vi "solar_cfg Write (Str).vi"(0 "Config Refnum":refnum<data-value>, 1 "Section":string, 2 "Comment":string, 5 "Key":string, 7 "Value in":string, 9 "Add Quotes? (T)":bool=TRUE, 11 "error in (no error)":errorcluster) -> (4 "dup Config Refnum":refnum<data-value>, 10 "Found?":bool, 15 "error out":errorcluster)   [LabVIEW 2018]
doc: "Write a value associated with a key to a specified section in the configuration file. Set a Comment (#...) to add a description after the key's value.\n\n[Section]\nKey = \"Value\" #Comment"
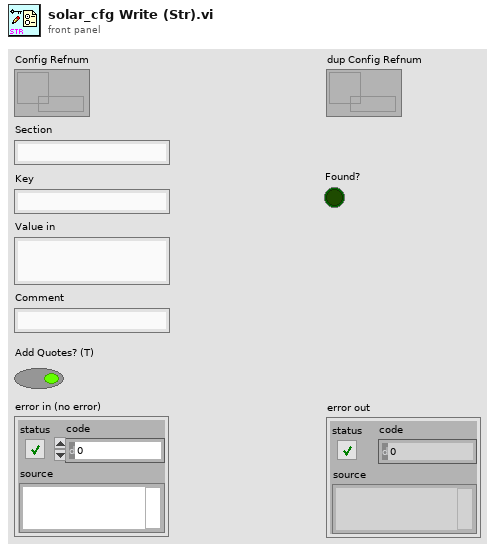
[diagram p1: front panel]
types:
  T1 = cluster{"Dirty":bool, "Semaphore":refnum<queue>, "Sections":cluster{"Section":string, "kvc":string[][]}[], "Path":path}
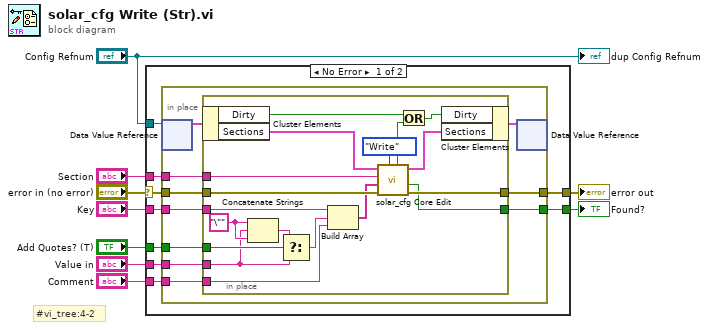
[diagram p0: block diagram]
diagram:
  # "#vi_tree:4-2"
  n1 = case shown="No Error" "error in (no error)" {
    selector: "error in (no error)" -> [w18 w47]
    tunnel: "Config Refnum" -> [w10 _]
    tunnel: "Key" -> [w16 _]
    tunnel: [w17 w47] -> w7
    tunnel: "Section" -> [w13 _]
    tunnel: "Value in" -> [w15 _]
    tunnel: "Comment" -> [w14 _]
    tunnel: [w12 _] -> w2
    tunnel: "Add Quotes? (T)" -> [w11 _]
    frame No Error {
      n2 = in-place {
        in-place-border: w18 -> [w28]
        in-place-border: [w27] -> w17
        in-place-border: w16 -> [w26]
        in-place-border: w15 -> [w25]
        in-place-border: w14 -> [w24]
        in-place-border: w13 -> [w23]
        in-place-border: [w20] -> w12
        in-place-border: w11 -> [w19]
        n3 = in-place-dvr #1(w10) -> (w22:T1)  [unwired: 1 out]
        n4 = in-place {
          in-place-border: w28 -> [w45]
          in-place-border: [w44] -> w27
          in-place-border: w26 -> [w43]
          in-place-border: w25 -> [w30]
          in-place-border: w24 -> [w42]
          in-place-border: w23 -> [w40]
          in-place-border: [w34] -> w20
          in-place-border: w19 -> [w33]
          w32 = "\"" ("string")
          n5 = in-place-cluster #2(w22) -> ("Dirty"=w39:bool, "Sections"=w36:cluster{"Section":string, "kvc":string[][]}[])
          n6 = Concatenate Strings(w32, w30, w32) -> (w31:string)
          n7 = Select(t=w31, s=w33, f=w30) -> (s? t:f=w29:string)
          n8 = Build Array(w43, w29, w42) -> (w41:string[])
          n9 = call "solar_cfg Core Edit.vi"("Action (Read)"=enum8{"Read", "Write", "Parse", "Build"}."Write", "error in (no error)"=w45, "kvc in"=w41, "Section/String in"=w40, "Sections in"=w36) -> ("error out"=w44:errorcluster, "Found?"=w34:bool, "Sections out"=w35:cluster{"Section":string, "kvc":string[][]}[], "Dirty?"=w37:bool)  [unwired: 2 in, 1 out]
          n10 = Or(x=w39, y=w37) -> (x .or. y?=w38:bool)
          n11 = in-place-cluster #2("Dirty"=w38, "Sections"=w35) -> (w21:T1)
        }
        n12 = in-place-dvr #1(w21) -> ()  [unwired: 2 out]
      }
    }
    frame Error {
    }
  }
  "error out" <- w7
  "Found?" <- w2
  "dup Config Refnum" <- "Config Refnum"
